vi "Spectral Measurements Express VI.vi"() -> ()   [LabVIEW 2022 SP3]
uses:
  <vilib>/express/express analysis/Spectral/Block/exnSpectralBlock spectral measurements RMS poly.vi
  <vilib>/express/express analysis/Spectral/Block/exnSpectralBlock spectral measurements RMS DDT.vi
  <vilib>/express/express analysis/Spectral/XNode/ExpressSpectralMeasurementsBlockNode.xnode
panel:
  in  "Frequency (Hz)":dbl(slide) scale=0.0..100.0
  in  "stop":bool
  out "Waveform Graph":dynamicdata(graph)
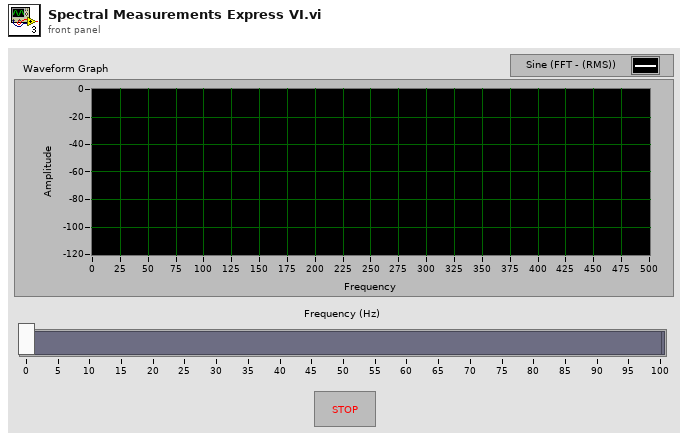
[diagram p1: front panel]
types:
  T1 = cluster{"averaging mode":u16, "weighting mode":u16, "number of averages":u32}
  T2 = cluster{"dB On (F)":bool, "unwrap phase (F)":bool, "convert to degree (F)":bool}
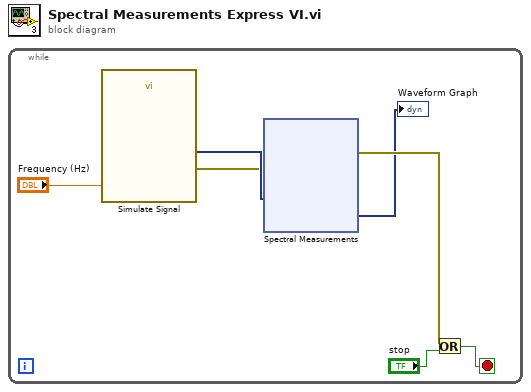
[diagram p0: block diagram]
diagram:
  n1 = while {
    stop <- w6 stop-if-true
    n2 = call "Simulate Signal"("Frequency"="Frequency (Hz)") -> ("Sine"=w4:dynamicdata, "error out"=w3:errorcluster)  [unwired: 13 in]
    n3 = xnode "Spectral Measurements"("Signals"=w4, "error in (no error)"=w3) -> ("FFT - (RMS)"=→"Waveform Graph":dynamicdata, "error out"=w2:errorcluster)  [unwired: 1 out]
    n4 = Or(x=w2, y="stop") -> (x .or. y?=w6:bool)
  }
